vi "Instance History.vi"(0 "Instance Data Array in":T1[](array[typedef]), 1 "Selected Instance":string, 2 "Class Data":refnum<class "Arithemetic Operation.lvclass">, 3 "Error In":errorcluster) -> (7 "Instance Data Array out":T1[](array[typedef]), 10 "Error Out":errorcluster)   [LabVIEW 2023, in "Arithemetic Operation.lvclass"]
uses:
  Arithemetic Operation.lvclass
  Typedef/Class Data.ctl
  Arithemetic Operation.lvclass/Arithemetic Operation.ctl
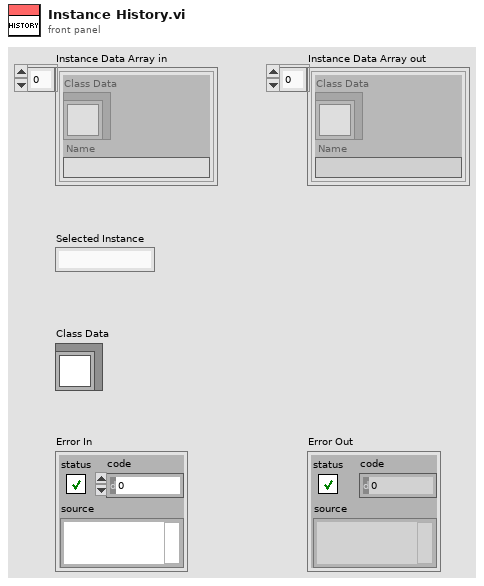
[diagram p1: front panel]
types:
  T1 = typedef "Class Data.ctl" = cluster{"Class Data":refnum<class "Arithemetic Operation.lvclass">, "Name":string}
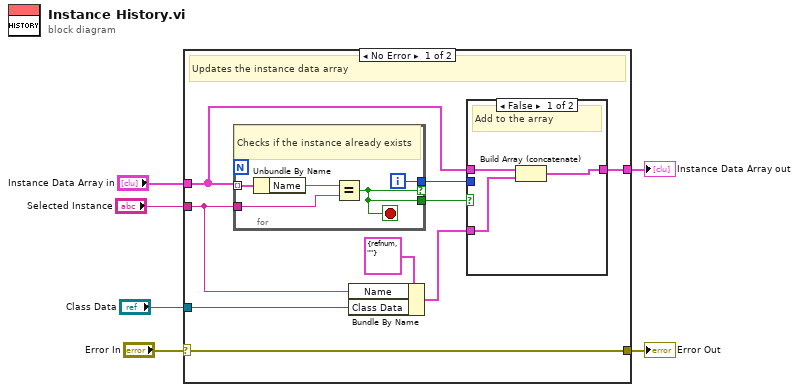
[diagram p0: block diagram]
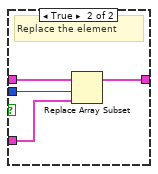
[diagram p2: hidden frame]
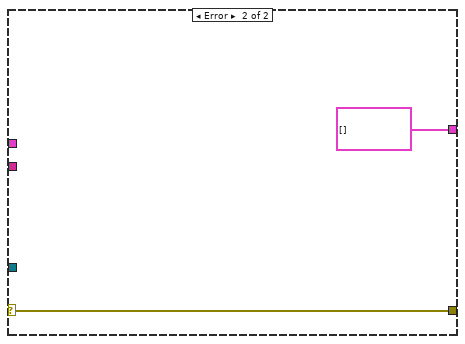
[diagram p3: hidden frame]
diagram:
  n1 = case shown="No Error" "Error In" {
    selector: "Error In" -> [w15 w29]
    tunnel: [w15 w29] -> w5
    tunnel: [w10 T1[] [] ("Instance Data Array in")] -> w4
    tunnel: "Class Data" -> [w9 _]
    tunnel: "Selected Instance" -> [w8 _]
    tunnel: "Instance Data Array in" -> [w7 _]
    frame No Error {
      # "Updates the instance data array"
      n2 = for {
        tunnel: w7 -> [w27] mode=indexing
        tunnel: w8 -> [w25]
        tunnel: [w24] -> w13 if=w23
        tunnel: [w23] -> w12
        i -> [w24]
        stop <- w23 stop-if-true
        # "Checks if the instance already exists"
        n3 = Unbundle By Name(w27) -> ("Name"=w26:string)
        n4 = Equal?(x=w26, y=w25) -> (x = y?=w23:bool)
      }
      n5 = Bundle By Name(cluster=T1 {"Class Data"=refnum, "Name"=""}, "Name"=w8, "Class Data"=w9) -> (w14:T1)
      n6 = case shown="False" w12 {
        tunnel: w13 -> [_ w22]
        tunnel: w7 -> [w18 w21]
        tunnel: w14 -> [w17 w20]
        tunnel: [w16 w19] -> w10
        frame False {
          # "Add to the array"
          n7 = Build Array (concatenate)(w18, w17) -> (w16:T1[])
        }
        frame True {
          # "Replace the element"
          n8 = Replace Array Subset(array=w21, new element=w20, index=w22) -> (w19:T1[])
        }
      }
    }
    frame Error {
    }
  }
  "Error Out" <- w5
  "Instance Data Array out" <- w4
